vi "Vernier pH meter v1_0.vi"() -> (0 "pH":dbl(knob) caption="Scaled Single Value" scale=0.0..14.0 scale format="%#.2f")   [LabVIEW 2012]
panel:
  out "Waveform Chart":dbl(graph) caption="pH Strip Chart"
  out "mean":dbl=4.307536760046787 format="%0.2f"
  in  "Offset":dbl=-0.14 min=-1.0 max=1.0 step=0.01 format="%.2f"
  # "Using the Vernier USB interface for the pH electrode here. The Venier drivers are not very robust/stable. If you see a NaN value displayed, the only option is to quit Labview and relauch the VI."
  # "An extremely simple diagnostic VI.\nUse it to check pH readings.\nAnd run it in the continous mode."
  # "To save offset:\n1) Right Click Offset value\n2) Highlight \"Data Operation\"\n3) Click make \"Make Current Value Default"
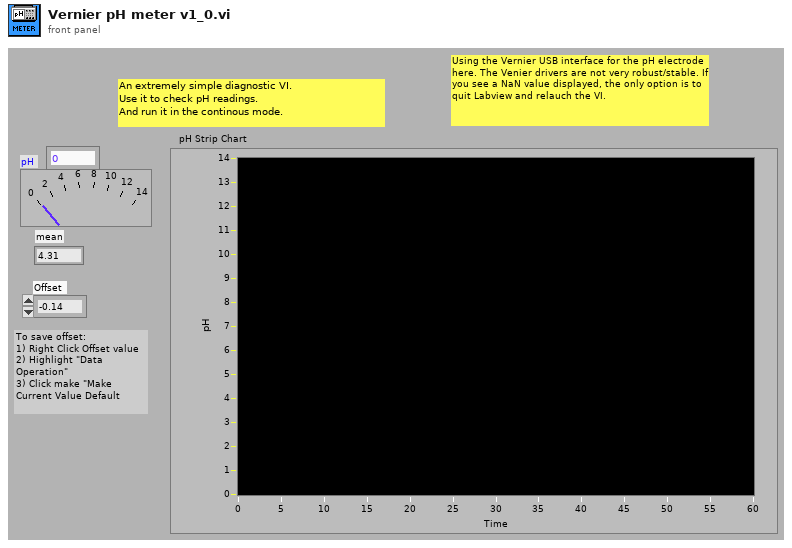
[diagram p1: front panel]
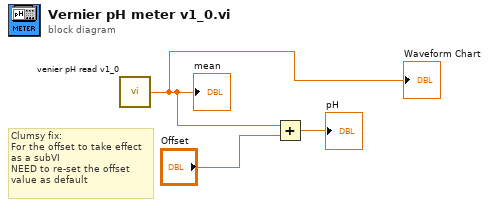
[diagram p0: block diagram]
diagram:
  # "Clumsy fix:\nFor the offset to take effect as a subVI\nNEED to re-set the offset value as default"
  n1 = call "venier pH read v1_0.vi"() -> ("mean"=w1:dbl)  [unwired: 2 in]
  "mean" <- w1
  "Waveform Chart" <- w1
  n2 = Add(x=w1, y="Offset") -> (x+y=→"pH":dbl)
